vi "MouseReadCore_subvi.vi"(10 "Pane":refnum<vi>, 11 "VI in":refnum<vi>) -> (1 "Vertical":i32, 2 "Mouse Y Abs":i32, 3 "Horizontal":i32, 4 "Mouse X Rel":i32, 5 "Mouse X Abs":i32, 6 "Mouse Y Rel":i32)   [LabVIEW 2019]
uses:
  <vilib>/Utility/inputDevices.llb/mouseAcquire.vi
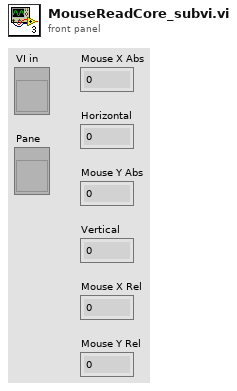
[diagram p1: front panel]
types:
  T1 = typedef "LVRectTypeDef.ctl" = cluster{"Left":i16, "Top":i16, "Right":i16, "Bottom":i16}
  T2 = typedef "LVPointTypeDef.ctl" = cluster{"Horizontal":i16, "Vertical":i16}
  T3 = cluster{"Horizontal":i32, "Vertical":i32, "Scrolling":i32}
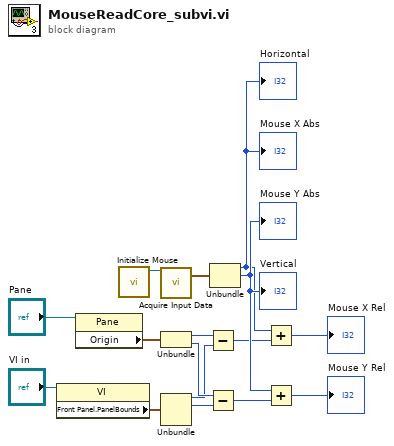
[diagram p0: block diagram]
diagram:
  n1 = property class="VI"(reference="VI in") -> ("Front Panel.PanelBounds"=w3:T1)  [unwired: 1 in, 2 out]
  n2 = property class="Pane"(reference="Pane") -> ("Origin"=w5:T2)  [unwired: 1 in, 2 out]
  n3 = call <vilib>:"Initialize Mouse.vi"() -> ("device ID"=w2:refnum<k1>)  [unwired: 10 in, 1 out]
  n4 = call-poly <vilib>:"Acquire Input Data.vi"("device ID"=w2) -> ("axis info"=w1:T3)  [unwired: 15 in, 3 out]
  n5 = Unbundle(w5) -> ("Horizontal"=w7:i16, "Vertical"=w9:i16)
  n6 = Unbundle(w3) -> ("Left"=w8:i16, "Top"=w10:i16)  [unwired: 2 out]
  n7 = Subtract(x=w7, y=w8) -> (x-y=w11:i16)
  n8 = Subtract(x=w9, y=w10) -> (x-y=w14:i16)
  n9 = Unbundle(w1) -> ("Horizontal"=w12:i32, "Vertical"=w15:i32)  [unwired: 1 out]
  "Mouse X Abs" <- w12
  "Mouse Y Abs" <- w15
  "Vertical" <- w15
  "Horizontal" <- w12
  n10 = Add(x=w12, y=w11) -> (x+y=→"Mouse X Rel":i32)
  n11 = Add(x=w15, y=w14) -> (x+y=→"Mouse Y Rel":i32)
